vi "AggregateResults (Cluster).vi"(7 "Section":string, 8 "error in (no error)":errorcluster, 10 "Value":variant, 11 "Pips in":refnum<class "Pips.lvclass">) -> (0 "error out":errorcluster, 3 "Pips out":refnum<class "Pips.lvclass">)   [LabVIEW 2021, in "Bananas.lvlib" / "Pips.lvclass"]
doc: "Accepts any type.\n\nIf of type Cluster, the Section field defaults to the cluster name. If the cluster name is empty, it will be marked as \"uncategorized\". Each element of the cluster will use the label as the key. If unnamed, they will be labeled element0..elementN-1\n\nIf of any type other than cluster, the Section field must be provided, otherwise it will be marked as \"uncategorized\". The Value label will become the key. If no label is found, it will be skipped."
uses:
  Pips.lvclass
  <vilib>/LabVIEW Open Source Project/Data Manipulation/TypeDescriptor/TypeDescriptor_GetType.vi
  <vilib>/LabVIEW Open Source Project/Data Manipulation/TypeDescriptor/TypeDescriptor_GetName.vi
  <vilib>/LabVIEW Open Source Project/Data Manipulation/TypeDescriptor/TypeDescriptor_GetPString.vi
  <vilib>/Utility/GetType.llb/Get Type Code from I16 Array And Pos.vi
  <vilib>/LabVIEW Open Source Project/Data Manipulation/Variant/OpenVariant.lvlib
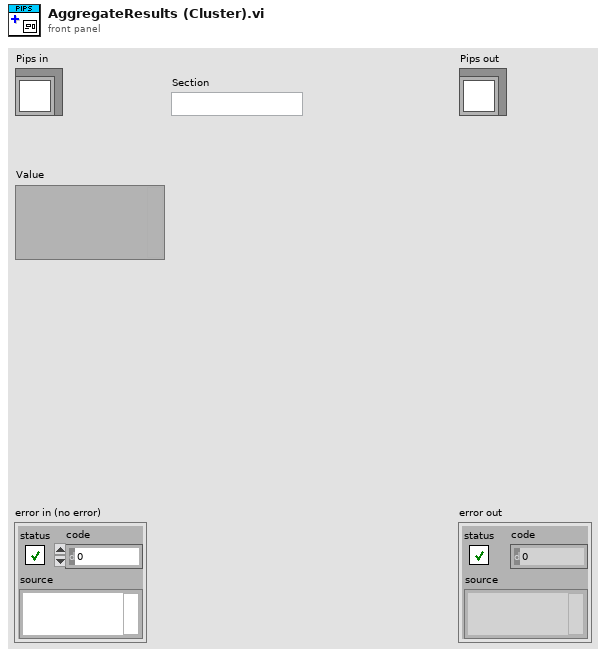
[diagram p1: front panel]
types:
  T1 = typedef "Type Enum.ctl" = enum8{"Void", "I8", "I16", "I32", "I64", "U8", "U16", "U32", "U64", "Single Float", "Double Float", "Extended Float", "Single Complex", "Double Complex", "Extended Complex", "Enum I8 NEVER", "Enum I16 NEVER", "Enum I32 NEVER", "Enum I64 NEVER", "Enum U8", "Enum U16", "Enum U32", "Enum U64", "Single Float With Unit", "Double Float With Unit", "Extended Float With Unit", "Single Complex With Unit", "Double Complex With Unit", "Extended Complex With Unit", "boolU16", "Boolean", "String", "Handle", "Path", "Picture", "C String", "Pascal String", "Tag", "SubString", "Array", "SubArray", "Cluster", "Numeric Cluster", "Variant", "LV Variant", "Measure Data (waveform)", "Refnum", "ExtData", "function", "Typedef", "Poly VI", "bad wire", "LabVIEW Class Instance"}
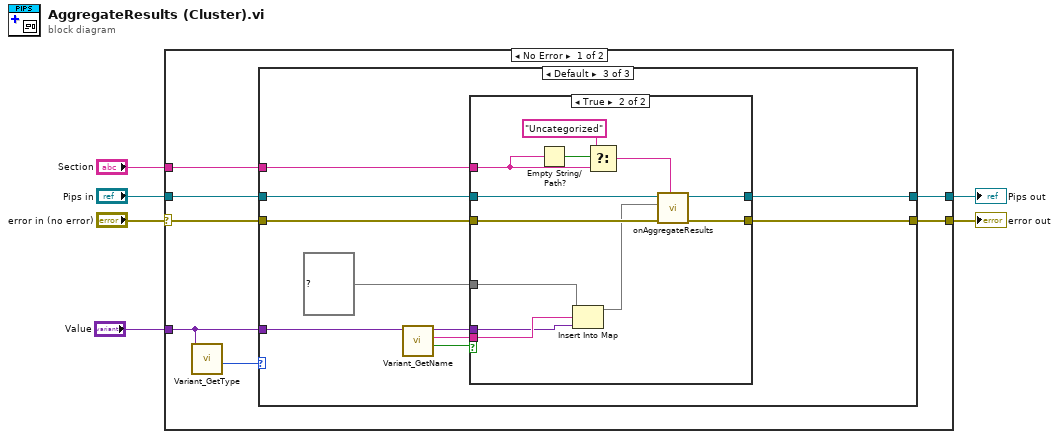
[diagram p0: block diagram]
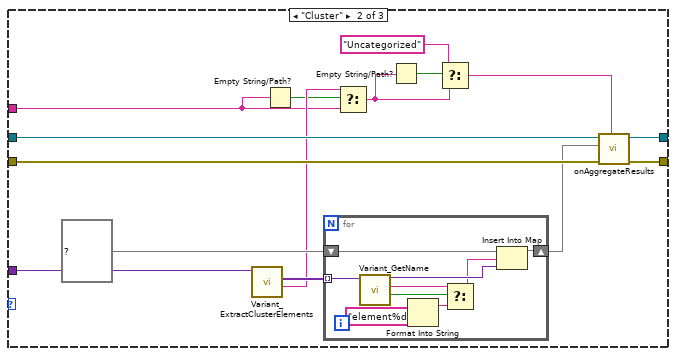
[diagram p3: hidden frame]
diagram:
  n1 = case shown="No Error" "error in (no error)" {
    selector: "error in (no error)" -> [w10 w66]
    tunnel: [w11 w66] -> w5
    tunnel: [w12 w65] -> w3
    tunnel: "Pips in" -> [w13 w65]
    tunnel: "Value" -> [w8 _]
    tunnel: "Section" -> [w9 _]
    frame No Error {
      n2 = call <vilib>:"Variant_GetType.vi"("Variant"=w8) -> ("Type Enum"=w7:T1)  [unwired: 8 in, 2 out]
      n3 = case shown="Default" w7 {
        tunnel: w13 -> [w15 w30 w50]
        tunnel: [w15 w29 w49] -> w12
        tunnel: [w14 w28 w48] -> w11
        tunnel: w10 -> [w14 w27 w47]
        tunnel: w9 -> [_ w18 w42]
        tunnel: w8 -> [_ w21 w44]
        frame "Void" {
        }
        frame "Cluster" {
          n4 = call <vilib>:"Variant_ExtractClusterElements.vi"("Cluster"=w21) -> ("name"=w24:string, "Elements"=w26:variant[])  [unwired: 8 in, 1 out]
          n5 = Empty String/Path?(string/path=w18) -> (empty?=w22:bool)
          n6 = for {
            tunnel: w26 -> [w40] mode=indexing
            shift-right: [w38] -> w23
            shift-left: map{string, variant} {} ("Results") -> [w39]
            i -> [w33]
            n7 = call <vilib>:"Variant_GetName.vi"("Variant"=w40) -> ("found"=w36:bool, "Name"=w35:string, "Variant dup"=w37:variant)  [unwired: 8 in]
            n8 = Format Into String(format string="element%d", w33) -> (resulting string=w32:string)  [unwired: 2 in, 1 out]
            n9 = Select(t=w35, s=w36, f=w32) -> (s? t:f=w34:string)
            n10 = Insert Into Map(map in=w39, key=w34, value=w37) -> (map out=w38:map{string, variant})  [unwired: 2 out]
          }
          n11 = Select(t=w24, s=w22, f=w18) -> (s? t:f=w17:string)
          n12 = Empty String/Path?(string/path=w17) -> (empty?=w20:bool)
          n13 = Select(t="Uncategorized", s=w20, f=w17) -> (s? t:f=w16:string)
          n14 = call-dynamic "onAggregateResults.vi"("Section"=w16, "error in (no error)"=w27, "Results"=w23, "Pips in"=w30) -> ("error out"=w28:errorcluster, "Pips out"=w29:refnum<class "Pips.lvclass">)  [unwired: 6 in]
        }
        frame Default {
          n15 = call <vilib>:"Variant_GetName.vi"("Variant"=w44) -> ("found"=w41:bool, "Name"=w45:string, "Variant dup"=w43:variant)  [unwired: 8 in]
          n16 = case shown="True" w41 {
            tunnel: w50 -> [w52 w64]
            tunnel: [w52 w63] -> w49
            tunnel: [w51 w62] -> w48
            tunnel: w47 -> [w51 w61]
            tunnel: map{string, variant} {} ("Results") -> [_ w60]
            tunnel: w45 -> [_ w56]
            tunnel: w43 -> [_ w55]
            tunnel: w42 -> [_ w54]
            frame False {
            }
            frame True {
              n17 = Empty String/Path?(string/path=w54) -> (empty?=w57:bool)
              n18 = Insert Into Map(map in=w60, key=w56, value=w55) -> (map out=w58:map{string, variant})  [unwired: 2 out]
              n19 = Select(t="Uncategorized", s=w57, f=w54) -> (s? t:f=w59:string)
              n20 = call-dynamic "onAggregateResults.vi"("Section"=w59, "error in (no error)"=w61, "Results"=w58, "Pips in"=w64) -> ("error out"=w62:errorcluster, "Pips out"=w63:refnum<class "Pips.lvclass">)  [unwired: 6 in]
            }
          }
        }
      }
    }
    frame Error {
    }
  }
  "error out" <- w5
  "Pips out" <- w3
